vi "MoveToStrip.vi"(6 "Single Needle":bool, 8 "Error In":errorcluster, 9 "Strip No.":u16, 10 "Region":u16, 11 "ProbeStationControl in":refnum<class "ProbeStationControl.lvclass">) -> (0 "Error Out":errorcluster, 2 "Z [µm]":i32, 3 "ProbeStationControl out":refnum<class "ProbeStationControl.lvclass">)   [LabVIEW 2019]
doc: "Move to specified strip index and touch down probe."
uses:
  InstrControl/ProbeStationControl/ProbeStationControl.lvclass
  ProbePlanParams.vi
panel:
  out "time3":u32
  out "time2":u32
  out "time1":u32
  out "previous Z [µm]":i32
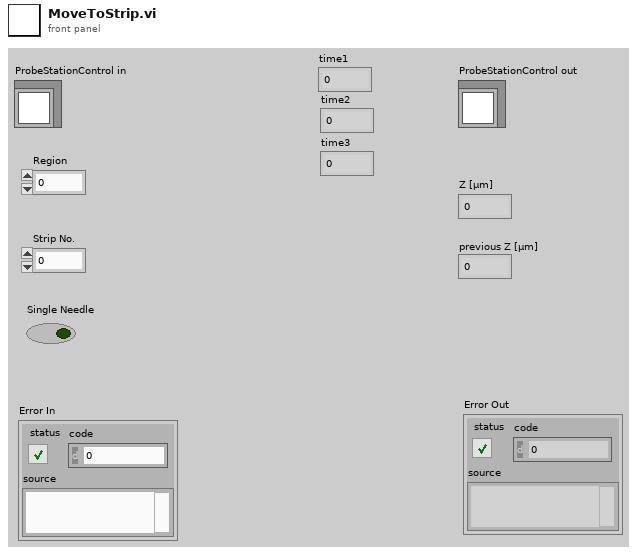
[diagram p1: front panel]
types:
  T1 = cluster{"Strip Number OUT":i32, "X0":i32, "Y0":i32, "X1":i32, "Y1":i32, "Xref":dbl, "Yref":dbl, "ProbePlan type":u32, "Inner pads offset":ext, "Outer pads offset":ext, "l_inner":ext, "l_outer":ext, "strip numbering":u16, "Device Orientation":ext, "Stagger offset":i32, "Yoffset":dbl, "Strip pitch":dbl, "Fiducail separation":dbl, "Radius":ext, "Relative strip angles":dbl, "Probeplan description":string, "ProbePlan array":cluster{"Region":string, "ProbePoints":cluster{"X":dbl, "Y":dbl, "Label":string, "CardViable?":bool}[]}[], "Test ProbePoints":cluster{"Regions Enabled":bool[], "From index":u32[], "To index":u32[]}}
  T2 = cluster{"Region":string, "ProbePoints":cluster{"X":dbl, "Y":dbl, "Label":string, "CardViable?":bool}[]}[]
  T3 = cluster{"Region":string, "ProbePoints":cluster{"X":dbl, "Y":dbl, "Label":string, "CardViable?":bool}[]}
  T4 = cluster{"X":dbl, "Y":dbl, "Label":string, "CardViable?":bool}[]
  T5 = cluster{"X":dbl, "Y":dbl, "Label":string, "CardViable?":bool}
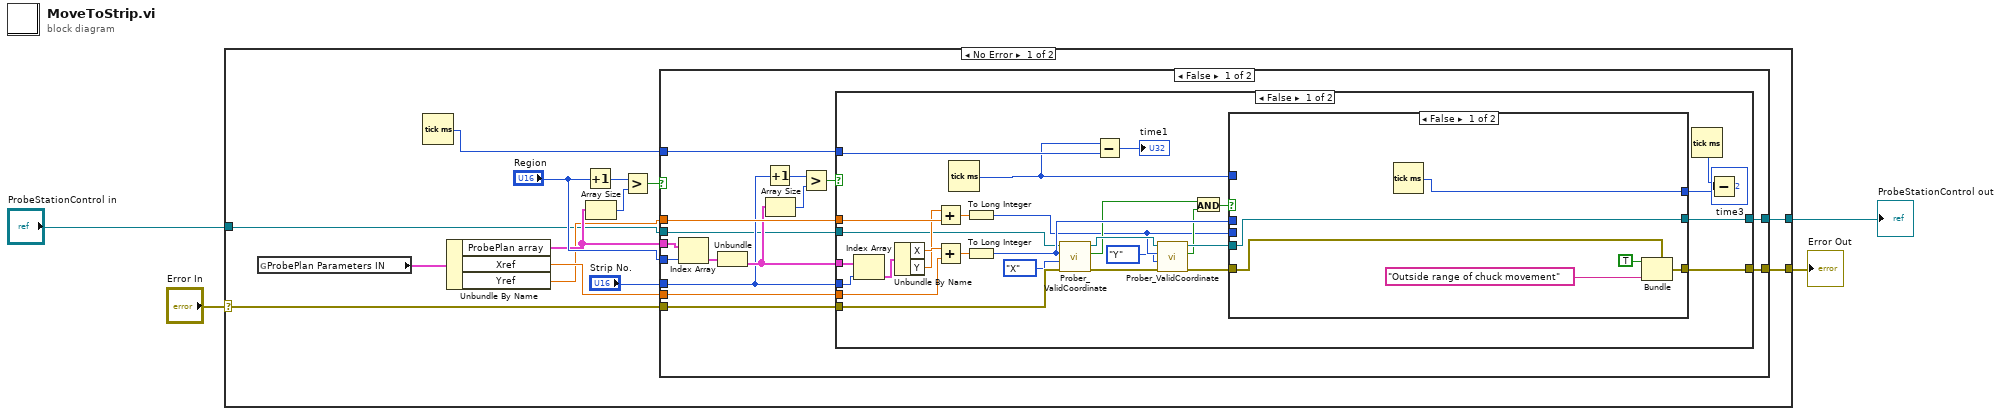
[diagram p0: block diagram]
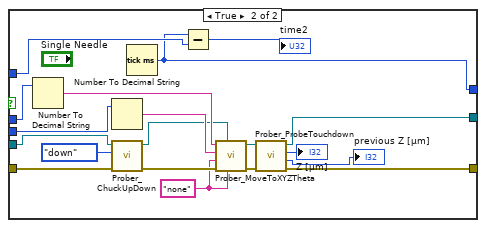
[diagram p2: hidden frame]
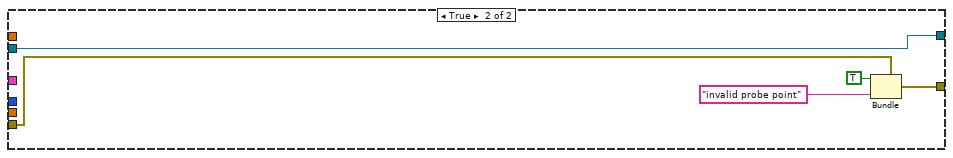
[diagram p3: hidden frame]
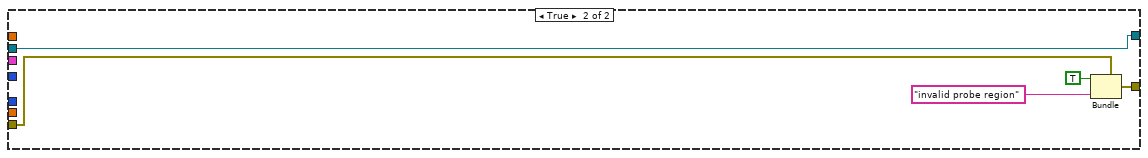
[diagram p4: hidden frame]
diagram:
  n1 = case shown="No Error" "Error In" {
    selector: "Error In" -> [w13 w99]
    tunnel: [w18 w99] -> w4
    tunnel: "ProbeStationControl in" -> [w7 w100]
    tunnel: [w8 w100] -> w1
    frame No Error {
      n2 = global read "ProbePlanParams.vi" "ProbePlan Parameters IN"() -> (w12:T1)
      n3 = Tick Count (ms)() -> (millisecond timer value=w6:u32)
      n4 = Unbundle By Name(w12) -> ("ProbePlan array"=w11:T2, "Xref"=w10:dbl, "Yref"=w9:dbl)
      n5 = Increment(x="Region") -> (x+1=w5:u16)
      n6 = Array Size(array=w11) -> (size(s)=w15:i32)
      n7 = Greater?(x=w5, y=w15) -> (0:w14:bool)
      n8 = case shown="False" w14 {
        tunnel: w13 -> [w28 w98]
        tunnel: [w27 w97] -> w18
        tunnel: "Region" -> [w31 _]
        tunnel: "Strip No." -> [w22 _]
        tunnel: w11 -> [w32 _]
        tunnel: w9 -> [w25 _]
        tunnel: w10 -> [w24 _]
        tunnel: [w21 w94] -> w8
        tunnel: w7 -> [w20 w94]
        tunnel: w6 -> [w19 _]
        frame False {
          n9 = Index Array(array=w32, index=w31) -> (element=w33:T3)
          n10 = Unbundle(w33) -> ("ProbePoints"=w23:T4)  [unwired: 1 out]
          n11 = Increment(x=w22) -> (x+1=w29:u16)
          n12 = Array Size(array=w23) -> (size(s)=w30:i32)
          n13 = Greater?(x=w29, y=w30) -> (0:w26:bool)
          n14 = case shown="False" w26 {
            tunnel: w28 -> [w50 w92]
            tunnel: [w56 w91] -> w27
            tunnel: w25 -> [w63 _]
            tunnel: w24 -> [w62 _]
            tunnel: w23 -> [w61 _]
            tunnel: w22 -> [w60 _]
            tunnel: [w53 w89] -> w21
            tunnel: w20 -> [w51 w89]
            tunnel: w19 -> [w38 _]
            frame False {
              n15 = Index Array(array=w61, index=w60) -> (element=w59:T5)
              n16 = Unbundle By Name(w59) -> ("X"=w58:dbl, "Y"=w57:dbl)
              n17 = Add(x=w57, y=w63) -> (x+y=w54:dbl)
              n18 = Add(x=w58, y=w62) -> (x+y=w55:dbl)
              n19 = Tick Count (ms)() -> (millisecond timer value=w37:u32)
              n20 = To Long Integer(number=w54) -> (32bit integer=w42:i32)
              n21 = To Long Integer(number=w55) -> (32bit integer=w52:i32)
              n22 = call-dynamic "Prober_ValidCoordinate.vi"("error in (no error)"=w50, "Axis"=enum16{"X", "Y", "Z", "Theta"}."X", "Coordinate IN"=w52, "ProbeStationControl in"=w51) -> ("error out"=w49:errorcluster, "Is Valid?"=w44:bool, "ProbeStationControl out"=w47:refnum<class "ProbeStationControl.lvclass">)  [unwired: 5 in]
              n23 = Subtract(x=w37, y=w38) -> (x-y=→"time1":u32)
              n24 = call-dynamic "Prober_ValidCoordinate.vi"("error in (no error)"=w49, "Axis"=enum16{"X", "Y", "Z", "Theta"}."Y", "Coordinate IN"=w42, "ProbeStationControl in"=w47) -> ("error out"=w48:errorcluster, "Is Valid?"=w45:bool, "ProbeStationControl out"=w46:refnum<class "ProbeStationControl.lvclass">)  [unwired: 5 in]
              n25 = And(x=w44, y=w45) -> (x .and. y?=w43:bool)
              n26 = case shown="False" w43 {
                tunnel: w48 -> [w67 w74]
                tunnel: [w66 w83] -> w56
                tunnel: w52 -> [_ w88]
                tunnel: w42 -> [_ w87]
                tunnel: [w65 w82] -> w53
                tunnel: w46 -> [w65 w75]
                tunnel: w37 -> [_ w72]
                tunnel: [w64 w70] -> w35
                frame False {
                  n27 = Tick Count (ms)() -> (millisecond timer value=w64:u32)
                  n28 = Bundle(cluster=w67, "status"=TRUE, "source"="Outside range of chuck movement") -> (w66:errorcluster)  [unwired: 1 in]
                }
                frame True {
                  w73 = "none"
                  n29 = Number To Decimal String(number=w88) -> (decimal integer string=w86:string)  [unwired: 1 in]
                  n30 = Number To Decimal String(number=w87) -> (decimal integer string=w85:string)  [unwired: 1 in]
                  n31 = call-dynamic "Prober_ChuckUpDown.vi"("error in (no error)"=w74, "Direction"=enum16{"up", "down"}."down", "ProbeStationControl in"=w75) -> ("error out"=w79:errorcluster, "ProbeStationControl out"=w80:refnum<class "ProbeStationControl.lvclass">)  [unwired: 6 in, 1 out]
                  n32 = Tick Count (ms)() -> (millisecond timer value=w70:u32)
                  n33 = Subtract(x=w70, y=w72) -> (x-y=→"time2":u32)
                  n34 = call-dynamic "Prober_MoveToXYZTheta.vi"("Theta location [mdeg]"=w73, "ProbeStationControl in"=w80, "error in (no error)"=w79, "Z location [µm]"=w73, "Y location [µm]"=w85, "X location [µm]"=w86) -> ("error out"=w84:errorcluster, "ProbeStationControl out"=w81:refnum<class "ProbeStationControl.lvclass">)  [unwired: 3 in, 1 out]
                  n35 = call-dynamic "Prober_ProbeTouchdown.vi"("error in (no error)"=w84, "ProbeStationControl in"=w81) -> ("error out"=w83:errorcluster, "previous Z [µm]"=→"previous Z [µm]":i32, "Z [µm]"=→"Z [µm]":i32, "ProbeStationControl out"=w82:refnum<class "ProbeStationControl.lvclass">)  [unwired: 6 in]
                }
              }
              n36 = Tick Count (ms)() -> (millisecond timer value=w36:u32)
              n37 = Subtract(x=w36, y=w35) -> (x-y=→"time3":u32)
            }
            frame True {
              n38 = Bundle(cluster=w92, "status"=TRUE, "source"="invalid probe point") -> (w91:errorcluster)  [unwired: 1 in]
            }
          }
        }
        frame True {
          n39 = Bundle(cluster=w98, "status"=TRUE, "source"="invalid probe region") -> (w97:errorcluster)  [unwired: 1 in]
        }
      }
    }
    frame Error {
    }
  }
  "Error Out" <- w4
  "ProbeStationControl out" <- w1
